vi "WLAN_SuperposedFrameBuild.vi"(6 "OFDMON":bool, 7 "Alpha":dbl min=0.0 max=1.0 step=0.05 format="%#_13g", 8 "error in (no error)":errorcluster, 9 "data in 2":i8[](array[numeric]) caption="input bit stream", 10 "Modulation parameter":T1, 11 "data in":i8[](array[numeric]) caption="input bit stream") -> (0 "error out":errorcluster, 3 "output array":cdb[](array[numeric]))   [LabVIEW 2022 SP3]
panel:
  in  "data in 3":i8[](array[numeric]) caption="input bit stream"
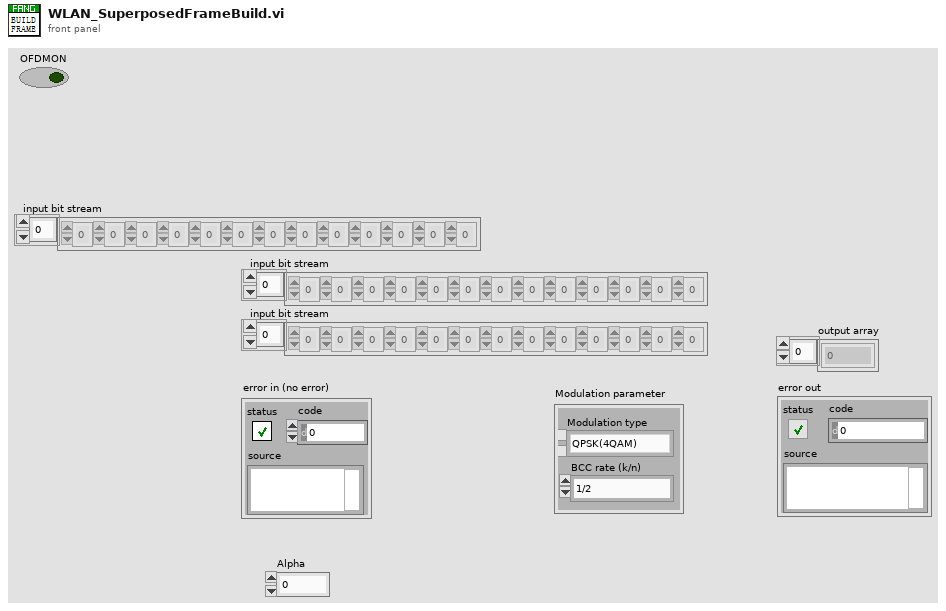
[diagram p1: front panel]
types:
  T1 = cluster{"Modulation type":enum16{"QPSK(4QAM)", "64QAM", "16QAM", "BPSK"}, "BCC rate (k/n)":enum16{"1/2", "2/3", "3/4"}}
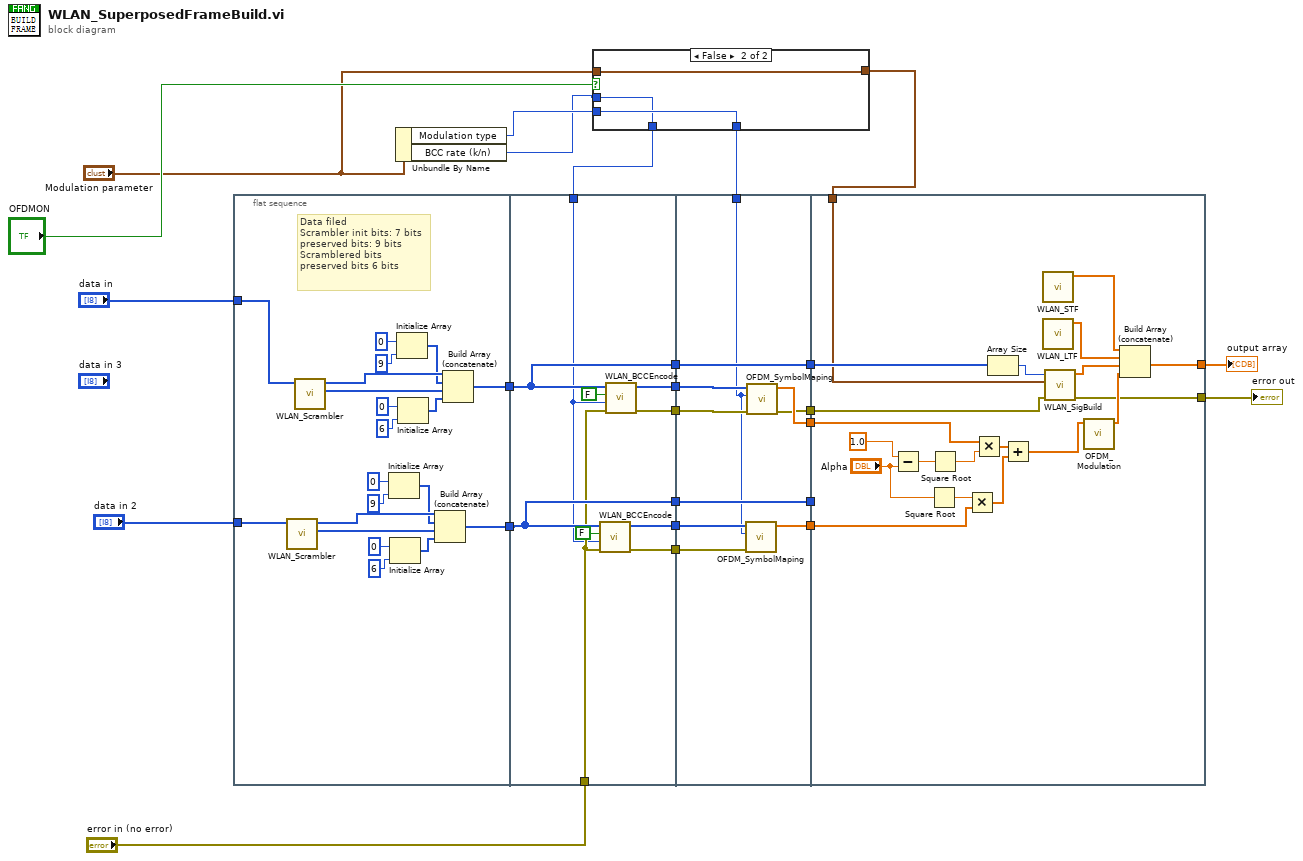
[diagram p0: block diagram]
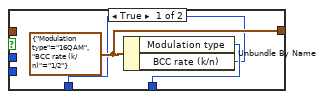
[diagram p2: hidden frame]
diagram:
  n1 = flat-sequence {
    tunnel: "data in" -> [w37]
    tunnel: [w36] -> w24
    tunnel: "data in 2" -> [w27]
    tunnel: [w26] -> w13
    tunnel: w24 -> [w52]
    tunnel: "error in (no error)" -> [w48]
    tunnel: [w54] -> w22
    tunnel: [w53] -> w21
    tunnel: w2 -> [w47]
    tunnel: [w52] -> w16
    tunnel: w13 -> [w50]
    tunnel: [w50] -> w12
    tunnel: [w49] -> w11
    tunnel: [w46] -> w9
    tunnel: w22 -> [w65]
    tunnel: w21 -> [w64]
    tunnel: w6 -> [w58]
    tunnel: [w63] -> w20
    tunnel: [w62] -> w19
    tunnel: w16 -> [w61]
    tunnel: [w61] -> w15
    tunnel: w12 -> [w59]
    tunnel: w11 -> [w60]
    tunnel: [w59] -> w10
    tunnel: w9 -> [w57]
    tunnel: [w56] -> w8
    tunnel: w4 -> [w83]
    tunnel: w20 -> [w68]
    tunnel: w19 -> [w78]
    tunnel: [w77] -> w18
    tunnel: [w76] -> w17
    tunnel: w15 -> [w85]
    tunnel: w10 -> [_]
    tunnel: w8 -> [w67]
    frame #0 {
      # "Data filed\nScrambler init bits: 7 bits\npreserved bits: 9 bits\nScramblered bits\npreserved bits 6 bits"
      n2 = call "WLAN_Scrambler.vi"("input bit stream"=w27) -> ("scrambled bits"=w31:i8[], "scrambler initial bit"=w35:i8[])  [unwired: 9 in]
      n3 = call "WLAN_Scrambler.vi"("input bit stream"=w37) -> ("scrambled bits"=w41:i8[], "scrambler initial bit"=w45:i8[])  [unwired: 9 in]
      n4 = Initialize Array(i8 0 ("element"), 9 ("dimension size")) -> (w34:i8[])
      n5 = Initialize Array(i8 0 ("element"), 6 ("dimension size")) -> (w28:i8[])
      n6 = Initialize Array(i8 0 ("element"), 9 ("dimension size")) -> (w44:i8[])
      n7 = Initialize Array(i8 0 ("element"), 6 ("dimension size")) -> (w38:i8[])
      n8 = Build Array (concatenate)(w35, w34, w31, w28) -> (w26:i8[])
      n9 = Build Array (concatenate)(w45, w44, w41, w38) -> (w36:i8[])
    }
    frame #1 {
      n10 = call "WLAN_BCCEncode.vi"("error in (no error)"=w48, "BCC rate (k/n)"=w47, "need add zeros?"=FALSE, "input bit stream"=w50) -> ("error out"=w46:errorcluster, "output bit stream 3"=w49:i8[])  [unwired: 6 in]
      n11 = call "WLAN_BCCEncode.vi"("error in (no error)"=w48, "BCC rate (k/n)"=w47, "need add zeros?"=FALSE, "input bit stream"=w52) -> ("error out"=w54:errorcluster, "output bit stream 3"=w53:i8[])  [unwired: 6 in]
    }
    frame #2 {
      n12 = call "OFDM_SymbolMaping.vi"("error in (no error)"=w57, "Modulation type"=w58, "input bit stream"=w60) -> ("symbols"=w56:cdb[])  [unwired: 7 in, 1 out]
      n13 = call "OFDM_SymbolMaping.vi"("error in (no error)"=w65, "Modulation type"=w58, "input bit stream"=w64) -> ("error out"=w62:errorcluster, "symbols"=w63:cdb[])  [unwired: 7 in]
    }
    frame #3 {
      n14 = Subtract(x=1.0, y="Alpha") -> (x-y=w70:dbl)
      n15 = Square Root(x="Alpha") -> (sqrt(x)=w74:dbl)
      n16 = Square Root(x=w70) -> (sqrt(x)=w72:dbl)
      n17 = Multiply(x=w74, y=w67) -> (x*y=w75:cdb[])
      n18 = Multiply(x=w68, y=w72) -> (x*y=w73:cdb[])
      n19 = Array Size(array=w85) -> (size(s)=w84:i32)
      n20 = Add(x=w73, y=w75) -> (x+y=w66:cdb[])
      n21 = call "WLAN_STF.vi"() -> ("STF"=w79:cdb[])  [unwired: 11 in]
      n22 = call "WLAN_LTF.vi"() -> ("LTF"=w80:cdb[])  [unwired: 11 in]
      n23 = call "WLAN_SigBuild.vi"("Data bit length"=w84, "Modulation parameter"=w83, "error in (no error)"=w78) -> ("symbols"=w81:cdb[], "error out"=w77:errorcluster)  [unwired: 6 in]
      n24 = call "OFDM_Modulation.vi"("Input sequence"=w66) -> ("Output sequence"=w82:cdb[])  [unwired: 10 in]
      n25 = Build Array (concatenate)(w79, w80, w81, w82) -> (w76:cdb[])
    }
  }
  n26 = Unbundle By Name("Modulation parameter") -> ("Modulation type"=w7:enum16{"QPSK(4QAM)", "64QAM", "16QAM", "BPSK"}, "BCC rate (k/n)"=w1:enum16{"1/2", "2/3", "3/4"})
  n27 = case shown="False" "OFDMON" {
    tunnel: w7 -> [_ w91]
    tunnel: [w88 w91] -> w6
    tunnel: [w87 w90] -> w4
    tunnel: "Modulation parameter" -> [_ w90]
    tunnel: [w86 w89] -> w2
    tunnel: w1 -> [_ w89]
    frame True {
      w87 = T1 {"Modulation type"=enum."16QAM", "BCC rate (k/n)"=enum."1/2"} ("Modulation parameter")
      n28 = Unbundle By Name(w87) -> ("Modulation type"=w88:enum16{"QPSK(4QAM)", "64QAM", "16QAM", "BPSK"}, "BCC rate (k/n)"=w86:enum16{"1/2", "2/3", "3/4"})
    }
    frame False {
    }
  }
  "output array" <- w17
  "error out" <- w18
